vi "Add Viewer.vi"(8 "error in (no error)":errorcluster, 10 "viewer":T1, 11 "Data Server Thread in":refnum<class "Data Server Thread.lvclass">) -> (0 "error out":errorcluster, 3 "Data Server Thread out":refnum<class "Data Server Thread.lvclass">)   [LabVIEW 2017, in "DSF Core.lvlib" / "Data Server Thread.lvclass"]
uses:
  Data Server Thread.lvclass
  Viewer Data.ctl
  Buffer/Buffer.lvclass
  Data Server Thread.lvclass/Data Server Thread.ctl
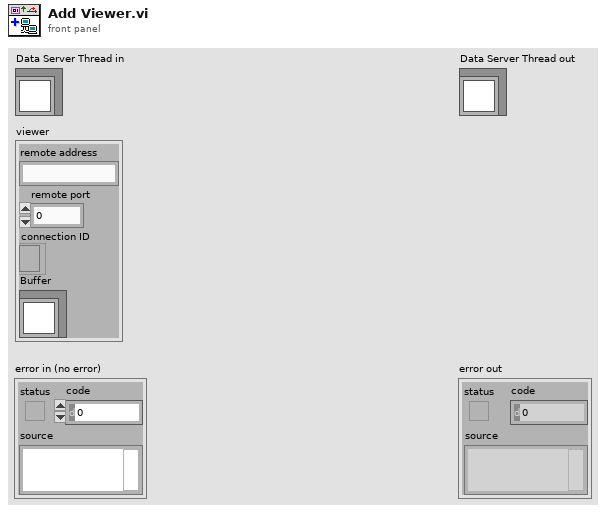
[diagram p1: front panel]
types:
  T1 = typedef "DSF Core.lvlib/Data Server Thread.lvclass/Viewer Data.ctl" = cluster{"remote address":string, "remote port":u16, "connection ID":refnum<k5>, "Buffer":refnum<class "Buffer.lvclass">}
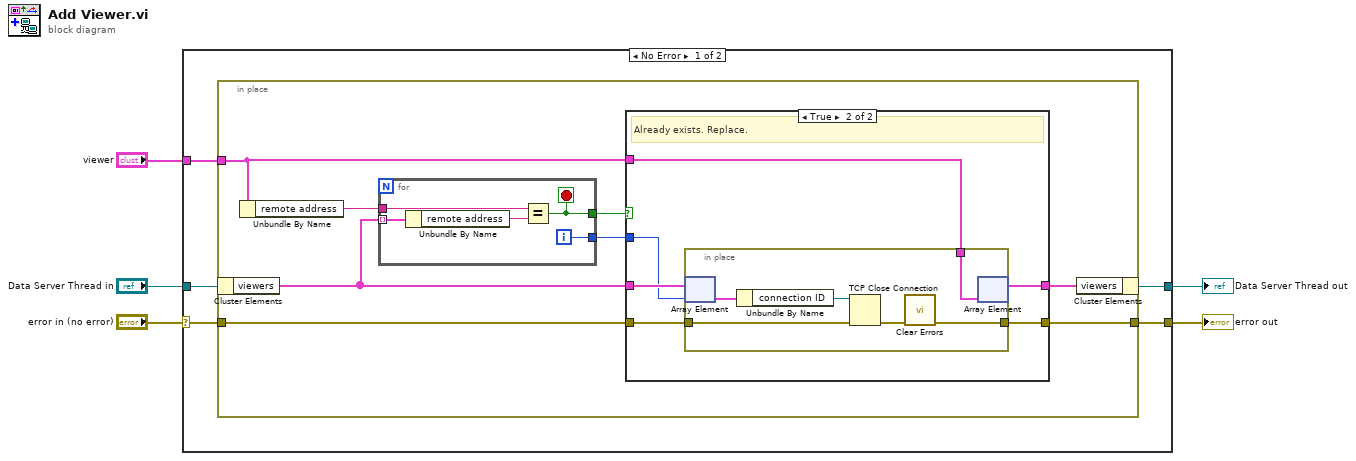
[diagram p0: block diagram]
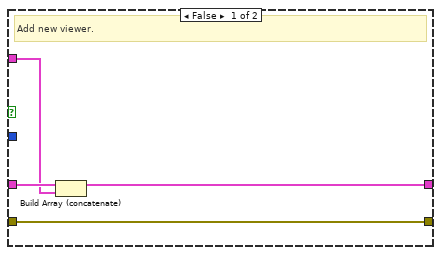
[diagram p2: hidden frame]
diagram:
  n1 = case shown="No Error" "error in (no error)" {
    selector: "error in (no error)" -> [w6 w41]
    tunnel: "Data Server Thread in" -> [w10 w40]
    tunnel: "viewer" -> [w9 _]
    tunnel: [w8 w41] -> w3
    tunnel: [w7 w40] -> w2
    frame No Error {
      n2 = in-place {
        in-place-border: w9 -> [w14]
        in-place-border: w6 -> [w12]
        in-place-border: [w11] -> w8
        n3 = in-place-cluster #1(w10) -> ("viewers"=w16:T1[])
        n4 = Unbundle By Name(w14) -> ("remote address"=w18:string)
        n5 = for {
          tunnel: w16 -> [w39] mode=indexing
          tunnel: w18 -> [w37]
          tunnel: [w36] -> w17
          tunnel: [w35] -> w13
          i -> [w35]
          stop <- w36 stop-if-true
          n6 = Unbundle By Name(w39) -> ("remote address"=w38:string)
          n7 = Equal?(x=w37, y=w38) -> (x = y?=w36:bool)
        }
        n8 = case shown="True" w17 {
          tunnel: w16 -> [w21 w24]
          tunnel: [w22 w28] -> w15
          tunnel: w14 -> [w20 w27]
          tunnel: w13 -> [_ w23]
          tunnel: w12 -> [w19 w26]
          tunnel: [w19 w25] -> w11
          frame False {
            # "Add new viewer."
            n9 = Build Array (concatenate)(w21, w20) -> (w22:T1[])
          }
          frame True {
            # "Already exists. Replace."
            n10 = in-place {
              in-place-border: [w29] -> w25
              in-place-border: w27 -> [w32]
              in-place-border: w26 -> [w31]
              n11 = in-place-array #2(w24, w23) -> (w34:T1)
              n12 = Unbundle By Name(w34) -> ("connection ID"=w33:refnum<k5>)
              n13 = TCP Close Connection(connection ID=w33, error in (no error)=w31) -> (error out=w30:errorcluster)  [unwired: 1 in, 1 out]
              n14 = call <vilib>:"Clear Errors.vi"("error in (no error)"=w30) -> ("error out"=w29:errorcluster)  [unwired: 5 in, 1 out]
              n15 = in-place-array #2(w32) -> (w28:T1[])  [unwired: 1 out]
            }
          }
        }
        n16 = in-place-cluster #1("viewers"=w15) -> (w7:refnum<class "Data Server Thread.lvclass">)
      }
    }
    frame Error {
    }
  }
  "error out" <- w3
  "Data Server Thread out" <- w2
